vi "generate table.vi"(5 "to cvt":refnum<vi>, 6 "View":enum32{"From Shared Memory", "To Shared Memory"}(ring), 7 "from cvt":refnum<vi>, 8 "error in":errorcluster, 9 "avail tags":refnum<vi>, 10 "engine configuration in":refnum<class "engine configuration.lvclass">, 11 "shm config in":refnum<class "Shared Memory configuration.lvclass">) -> (0 "error out":errorcluster, 2 "engine configuration out":refnum<class "engine configuration.lvclass">, 3 "shm config out":refnum<class "Shared Memory configuration.lvclass">)   [LabVIEW 2014, in "Shared Memory editor node.lvclass"]
uses:
  Shared Memory editor node.lvclass
  module/configuration/Shared Memory configuration.lvclass
  <vilib>/NI/Module Execution Interface/Engine Configuration/engine configuration.lvclass
  <vilib>/NI/Configuration Framework/serializable configuration/NISE_CEF_serializable configuration.lvclass/NISE_CEF_serializable configuration.ctl
  module/configuration/Shared Memory configuration.lvclass/Shared Memory configuration.ctl
  <vilib>/NI/Tag Bus/tag/tag descriptor.lvclass/tag descriptor.ctl
  <vilib>/NI/Tag Bus Module Framework/channel/channel classification.ctl
  <vilib>/NI/Tag Bus Module Framework/channel/TBM channel.lvclass/TBM channel.ctl
  <vilib>/NI/Module Execution Interface/Engine Configuration/engine configuration.lvclass/engine configuration.ctl
  <vilib>/NI/Tag Bus/tag/write tag name.vi
  <vilib>/NI/Tag Bus/tag/read tag name.vi
  <vilib>/NI/Tag Bus Module Framework/channel/Read channel classification.vi
  <vilib>/NI/Tag Bus/tag/read data type.vi
  <vilib>/Utility/LVClass/Get LV Class Name.vi
  <vilib>/NI/Configuration Framework/error generator/NISE_error generator.vi
  <vilib>/NI/Tag Bus Module Framework/channel/TBM channel.lvclass
  <vilib>/NI/Tag Bus/tag/tag descriptor.lvclass
  <vilib>/NI/Configuration Framework/serializable configuration/NISE_CEF_serializable configuration.lvclass
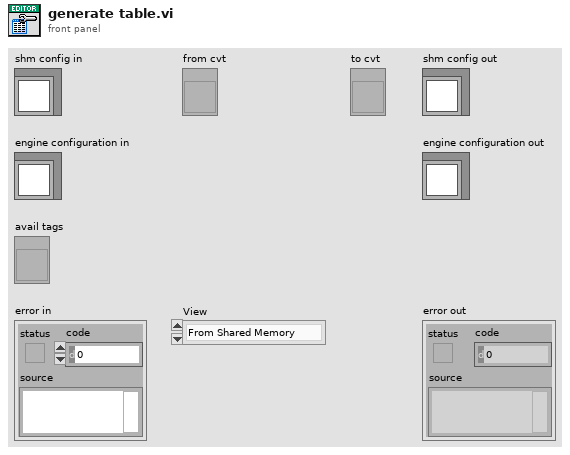
[diagram p1: front panel]
types:
  T1 = typedef "Shared Memory configuration.lvclass/Line.ctl" = cluster{"channel":refnum<class "TBM channel.lvclass">}
  T2 = typedef "tag bus.lvlib/tag descriptor.lvclass/Data Type.ctl" = enum16{"Double", "Single", "I64", "I32", "I16", "I8", "U64", "U32", "U16", "U8", "Boolean", "String", "Array of Double", "Array of Single", "Array of I64", "Array of I32", "Array of I16", "Array of I8", "Array of U64", "Array of U32", "Array of U16", "Array of U8", "Array of Boolean", "Array of String"}
  T3 = typedef "TBM channel.lvclass/channel classification.ctl" = enum16{"input data", "output data", "processing parameter", "processing result"}
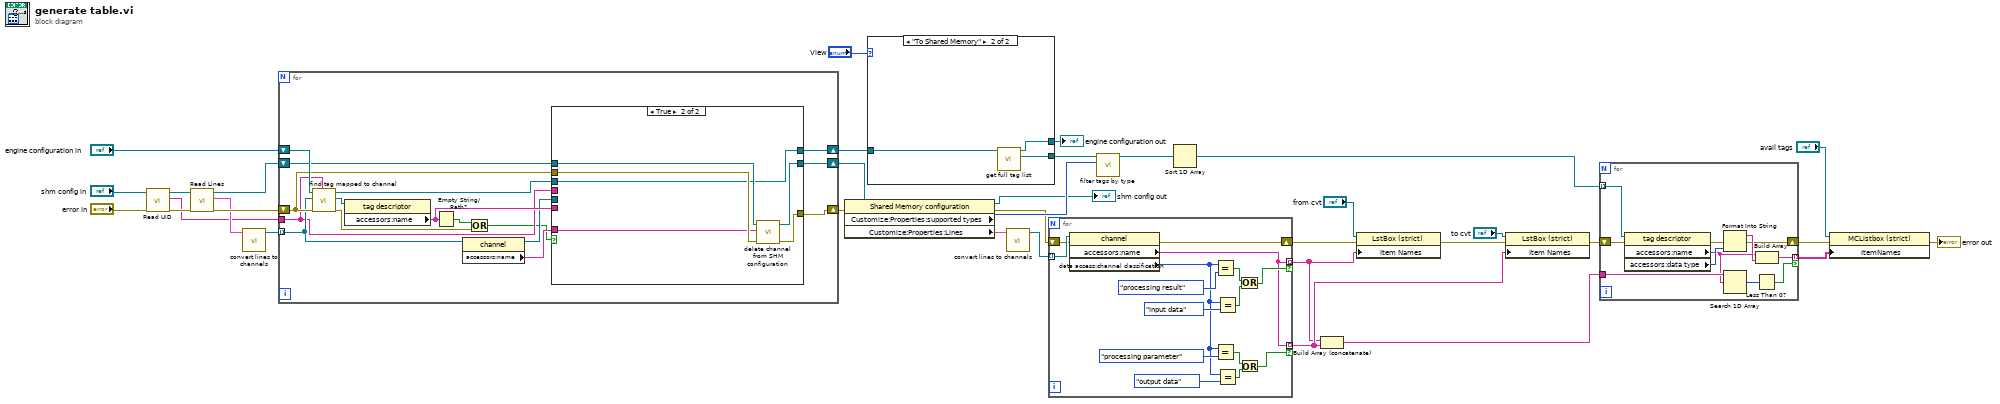
[diagram p0: block diagram]
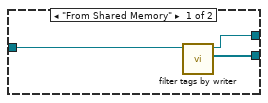
[diagram p2: hidden frame]
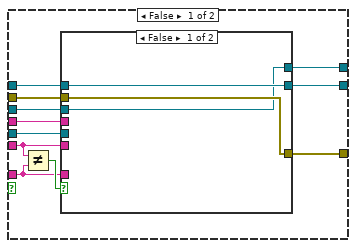
[diagram p3: hidden frame]
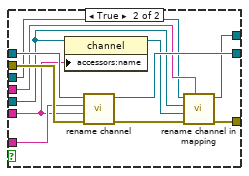
[diagram p4: hidden frame]
diagram:
  n1 = call <vilib>:"Read UID.vi"("error in"="error in", "configuration in"="shm config in") -> ("error out"=w9:errorcluster, "instance id"=w3:string, "configuration out"=w4:refnum<class "Shared Memory configuration.lvclass">)  [unwired: 7 in]
  n2 = call "Read Lines.vi"("error in"=w9, "Shared Memory configuration in"=w4) -> ("error out"=w6:errorcluster, "Lines"=w5:T1[], "Shared Memory configuration out"=w2:refnum<class "Shared Memory configuration.lvclass">)  [unwired: 7 in]
  n3 = call "convert lines to channels.vi"("Lines in"=w5) -> ("channels out"=w14:refnum<class "TBM channel.lvclass">[])  [unwired: 9 in, 1 out]
  n4 = for {
    tunnel: w14 -> [w42] mode=indexing
    shift-right: [w37] -> w25
    shift-left: "engine configuration in" -> [w51]
    shift-right: [w48] -> w35
    shift-left: w2 -> [w46]
    tunnel: w3 -> [w39]
    shift-right: [w47] -> w34
    shift-left: w6 -> [w45]
    n5 = call <vilib>:"find tag mapped to channel.vi"("owner"=w39, "error in"=w45, "channel"=w42, "engine configuration in"=w51) -> ("error out"=w44:errorcluster, "tag"=w50:refnum<class "tag descriptor.lvclass">, "engine configuration out"=w38:refnum<class "engine configuration.lvclass">)  [unwired: 5 in]
    n6 = property class="tag descriptor"(reference=w50) -> ("accessors:name"=w41:string)  [unwired: 1 in, 2 out]
    n7 = Empty String/Path?(string/path=w41) -> (empty?=w49:bool)
    n8 = property class="channel"(reference=w42) -> (reference out=w40:refnum<class "TBM channel.lvclass">, "accessors:name"=w43:string)  [unwired: 1 in, 1 out]
    n9 = Or(x=w49, y=w44) -> (x .or. y?=w36:bool)
    n10 = case shown="True" w36 {
      tunnel: [w59 w83] -> w48
      tunnel: [w62 w82] -> w47
      tunnel: w45 -> [w61 w81]
      tunnel: w46 -> [w60 w80]
      tunnel: w43 -> [w57 w79]
      tunnel: w41 -> [w56 _]
      tunnel: w40 -> [w55 _]
      tunnel: w39 -> [w54 _]
      tunnel: w38 -> [w53 w78]
      tunnel: [w52 w78] -> w37
      frame False {
        n11 = Not Equal?(x=w56, y=w57) -> (x != y?=w58:bool)
        n12 = case shown="False" w58 {
          tunnel: [w65 w72] -> w62
          tunnel: w61 -> [w65 w77]
          tunnel: w60 -> [w64 w76]
          tunnel: [w64 w75] -> w59
          tunnel: w57 -> [_ w74]
          tunnel: w56 -> [_ w71]
          tunnel: w55 -> [_ w70]
          tunnel: w54 -> [_ w68]
          tunnel: w53 -> [w63 w67]
          tunnel: [w63 w66] -> w52
          frame False {
          }
          frame True {
            n13 = property class="channel"(reference=w70, "accessors:name"=w71) -> (reference out=w69:refnum<class "TBM channel.lvclass">)  [unwired: 1 in, 1 out]
            n14 = call "rename channel.vi"("error in"=w77, "new name"=w71, "old name"=w74, "SHM configuration in"=w76) -> ("error out"=w73:errorcluster, "SHM configuration out"=w75:refnum<class "Shared Memory configuration.lvclass">)  [unwired: 6 in]
            n15 = call <vilib>:"rename channel in mapping.vi"("owner ID"=w68, "error in"=w73, "new channel"=w69, "old channel"=w70, "engine configuration in"=w67) -> ("error out"=w72:errorcluster, "engine configuration out"=w66:refnum<class "engine configuration.lvclass">)  [unwired: 5 in]
          }
        }
      }
      frame True {
        n16 = call "delete channel from SHM configuration.vi"("error in"=w81, "channel to delete"=w79, "SHM configuration in"=w80) -> ("error out"=w82:errorcluster, "SHM configuration out"=w83:refnum<class "Shared Memory configuration.lvclass">)  [unwired: 7 in]
      }
    }
  }
  n17 = property class="Shared Memory configuration"(reference=w35, error in=w34) -> (reference out=→"shm config out":refnum<class "Shared Memory configuration.lvclass">, error out=w32:errorcluster, "Customize:Properties:supported types"=w33:T2[], "Customize:Properties:Lines"=w13:T1[])
  n18 = case shown="\"To Shared Memory\"" "View" {
    tunnel: w25 -> [w86 w89]
    tunnel: [w85 w88] -> w24
    tunnel: [w84 w87] -> w15
    frame "From Shared Memory" {
      n19 = call <vilib>:"filter tags by writer.vi"("engine configuration in"=w86) -> ("tag list"=w85:refnum<class "tag descriptor.lvclass">[], "engine configuration out"=w84:refnum<class "engine configuration.lvclass">)  [unwired: 9 in]
    }
    frame "To Shared Memory" {
      n20 = call <vilib>:"get full tag list.vi"("engine configuration in"=w89) -> ("tag list"=w88:refnum<class "tag descriptor.lvclass">[], "engine configuration out"=w87:refnum<class "engine configuration.lvclass">)  [unwired: 9 in]
    }
  }
  "engine configuration out" <- w15
  n21 = call "convert lines to channels.vi"("Lines in"=w13) -> ("channels out"=w12:refnum<class "TBM channel.lvclass">[])  [unwired: 9 in, 1 out]
  n22 = for {
    tunnel: w12 -> [w104] mode=indexing
    shift-right: [w103] -> w20
    shift-left: w32 -> [w102]
    tunnel: [w97] -> w10 mode=indexing if=w90
    tunnel: [w97] -> w1 mode=indexing if=w98
    n23 = property class="channel"(reference=w104, error in=w102) -> (error out=w103:errorcluster, "accessors:name"=w97:string, "data access:channel classification"=w94:T3)  [unwired: 1 out]
    n24 = Equal?(x=w94, y=channel_classification."processing result") -> (x = y?=w99:bool)
    n25 = Equal?(x=w94, y=channel_classification."processing parameter") -> (x = y?=w91:bool)
    n26 = Equal?(x=w94, y=channel_classification."input data") -> (x = y?=w95:bool)
    n27 = Equal?(x=w94, y=channel_classification."output data") -> (x = y?=w92:bool)
    n28 = Or(x=w99, y=w95) -> (x .or. y?=w98:bool)
    n29 = Or(x=w91, y=w92) -> (x .or. y?=w90:bool)
  }
  n30 = call <vilib>:"filter tags by type.vi"("allowable types"=w33, "tags in"=w24) -> ("filtered tags"=w31:refnum<class "tag descriptor.lvclass">[])  [unwired: 9 in]
  n31 = Sort 1D Array(array=w31) -> (sorted array=w16:refnum<class "tag descriptor.lvclass">[])
  n32 = Build Array (concatenate)(w1, w10) -> (w17:string[])
  n33 = property class="LstBox (strict)"(reference="from cvt", error in=w20, "Item Names"=w1) -> (error out=w19:errorcluster)  [unwired: 1 out]
  n34 = property class="LstBox (strict)"(reference="to cvt", error in=w19, "Item Names"=w10) -> (error out=w30:errorcluster)  [unwired: 1 out]
  n35 = for {
    tunnel: w16 -> [w113] mode=indexing
    shift-right: [w110] -> w29
    shift-left: w30 -> [w112]
    tunnel: [w109] -> w28 mode=indexing if=w105
    tunnel: w17 -> [w108]
    n36 = property class="tag descriptor"(reference=w113, error in=w112) -> (error out=w111:errorcluster, "accessors:name"=w106:string, "accessors:data type"=w114:T2)  [unwired: 1 out]
    n37 = Format Into String(error in=w111, w114) -> (resulting string=w115:string, error out=w110:errorcluster)  [unwired: 2 in]
    n38 = Search 1D Array(1D array=w108, element=w106) -> (index of element=w107:i32)  [unwired: 1 in]
    n39 = Less Than 0?(x=w107) -> (x < 0?=w105:bool)
    n40 = Build Array(w106, w115) -> (w109:string[])
  }
  n41 = property class="MCListbox (strict)"(reference="avail tags", error in=w29, "ItemNames"=w28) -> (error out=→"error out":errorcluster)  [unwired: 1 out]
